vi "HyperTerm Data Decode.vi"(0 "Water Heater GEA2 Data in":T1 {"Hyperterminal Data"."CRC" format="%x"; "Hyperterminal Data"."Length" format="%x"; "Hyperterminal Data"."Command" format="%x"; "Hyperterminal Data"."Destination" format="%x"; "Hyperterminal Data"."Source" format="%x"}, 1 "Hex Array Out":string[](array[string]), 5 "Error In":errorcluster) -> (14 "Water Heater GEA2 Data out":T1 {"Hyperterminal Data"."CRC" format="%x"; "Hyperterminal Data"."Length" format="%x"; "Hyperterminal Data"."Command" format="%x"; "Hyperterminal Data"."Destination" format="%x"; "Hyperterminal Data"."Source" format="%x"}, 19 "Error Out":errorcluster)   [LabVIEW 2018]
uses:
  Type Definitions/GEA2 Commands WaterHeater GEA2 Data.ctl
  Type Definitions/GEA2 Commands Button Status.ctl
  Type Definitions/GEA2 Commands Status Query.ctl
  Type Definitions/GEA2 Commands Service Error Codes.ctl
panel:
  out "String":string
  out "T5(Ambient)":dbl
  out "T4(CompressorDischarge)":dbl
  out "T3B (EvapOut)":dbl
  out "T3A (EvapIN)":dbl
  out "T2 Tank Sensor":dbl
  out "Reason for Data Word 4":string
  out "Reason for Data Word 3":string
  out "Reason for Data Word 2":string
  out "Reason for Data Word 1":string
  out "Reason for last heating cycle termination":u16
  out "EEV Position (0-480)":u16
  out "Voltage (Volts)":u16
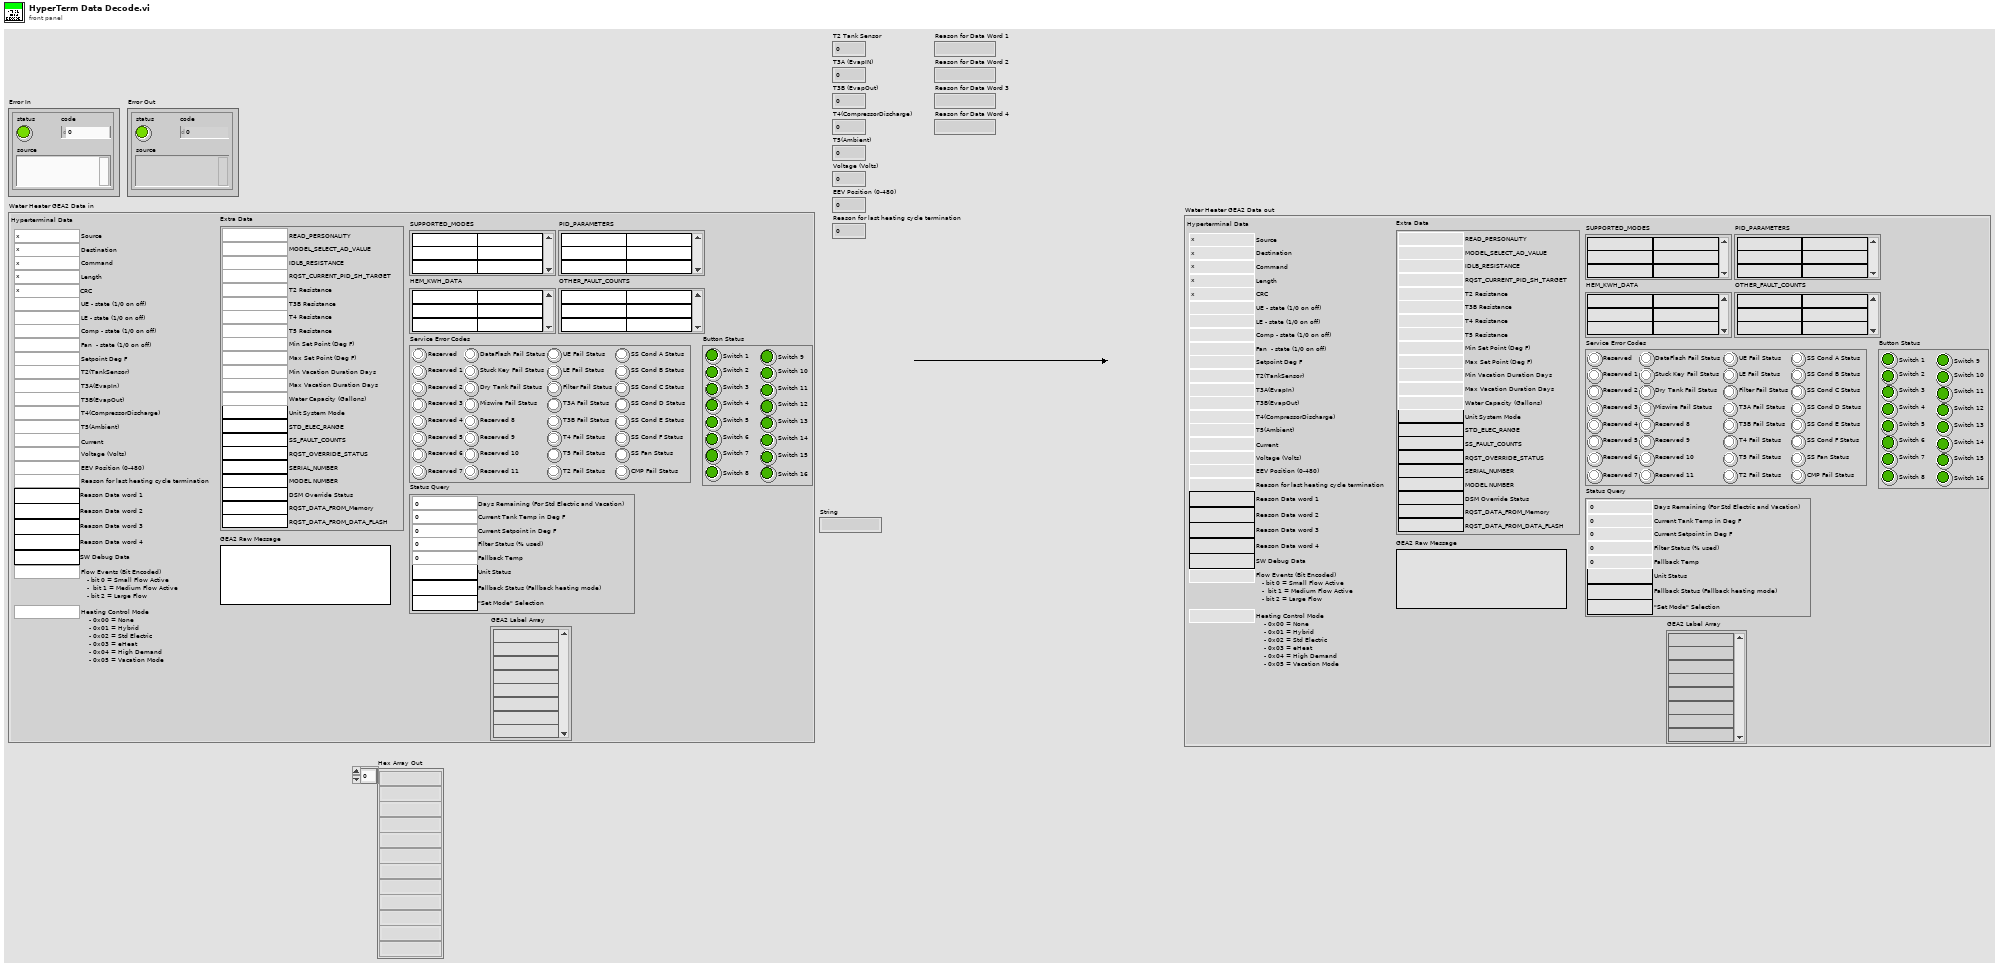
[diagram p1: front panel]
types:
  T1 = typedef "GEA2 Commands WaterHeater GEA2 Data.ctl" = cluster{"GEA2 Label Array":string[], "PID_PARAMETERS":string[][], "SUPPORTED_MODES":string[][], "Button Status":T2, "Status Query":T3, "Service Error Codes":T4, "HEM_KWH_DATA":string[][], "OTHER_FAULT_COUNTS":string[][], "GEA2 Raw Message":string, "Hyperterminal Data":cluster{"Source":u8, "Destination":u8, "Command":u8, "Length":u8, "CRC":u16, "UE - state (1/0 on off)":u8, "LE - state (1/0 on off)":u8, "Comp - state (1/0 on off)":u8, "Fan  - state (1/0 on off)":u8, "Setpoint Deg F":i32, "T2(TankSensor)":dbl, "T3A(EvapIn)":dbl, "T3B(EvapOut)":dbl, "T4(CompressorDischarge)":dbl, "T5(Ambient)":dbl, "Current":dbl, "Voltage (Volts)":u16, "EEV Position (0-480)":u16, "Reason for last heating cycle termination":u16, "Reason Data word 1":string, "Reason Data word 2":string, "Reason Data word 3":string, "Reason Data word 4":string, "SW Debug Data":string, "Flow Events (Bit Encoded)":u16, "Heating Control Mode":u16}, "Extra Data":cluster{"Water Capacity (Gallons)":u32, "Max Vacation Duration Days":u32, "Min Vacation Duration Days":u32, "Max Set Point (Deg F)":u32, "Min Set Point (Deg F)":u32, "T5 Resistance":u32, "T4 Resistance":u32, "T3B Resistance":u32, "T2 Resistance":u32, "STD_ELEC_RANGE":string, "SS_FAULT_COUNTS":string, "SERIAL_NUMBER":string, "READ_PERSONALITY":u8, "RQST_OVERRIDE_STATUS":string, "MODEL_SELECT_AD_VALUE":u32, "MODEL NUMBER":string, "IDLB_RESISTANCE":u32, "DSM Override Status":string, "RQST_DATA_FROM_Memory":string, "RQST_DATA_FROM_DATA_FLASH":string, "RQST_CURRENT_PID_SH_TARGET":u16, "Unit System Mode":string}}
  T2 = typedef "GEA2 Commands Button Status.ctl" = cluster{"Switch 1":bool, "Switch 2":bool, "Switch 3":bool, "Switch 4":bool, "Switch 5":bool, "Switch 6":bool, "Switch 7":bool, "Switch 8":bool, "Switch 9":bool, "Switch 10":bool, "Switch 11":bool, "Switch 12":bool, "Switch 13":bool, "Switch 14":bool, "Switch 15":bool, "Switch 16":bool}
  T3 = typedef "GEA2 Commands Status Query.ctl" = cluster{"Days Remaining (For Std Electric and Vacation)":u8, "Unit Status":string, "Current Tank Temp in Deg F":u8, "Current Setpoint in Deg F":u8, "Filter Status (% used)":u8, "Fallback Status (Fallback heating mode)":string, "Fallback Temp":u8, "\"Set Mode\" Selection":string}
  T4 = typedef "GEA2 Commands Service Error Codes.ctl" = cluster{"Reserved":bool, "Reserved 1":bool, "Reserved 2":bool, "Reserved 3":bool, "Reserved 4":bool, "Reserved 5":bool, "Reserved 6":bool, "Reserved 7":bool, "DataFlash Fail Status":bool, "Stuck Key Fail Status":bool, "Dry Tank Fail Status":bool, "Miswire Fail Status":bool, "Reserved 8":bool, "Reserved 9":bool, "Reserved 10":bool, "Reserved 11":bool, "UE Fail Status":bool, "LE Fail Status":bool, "Filter Fail Status":bool, "T3A Fail Status":bool, "T3B Fail Status":bool, "T4 Fail Status":bool, "T5 Fail Status":bool, "T2 Fail Status":bool, "SS Cond A Status":bool, "SS Cond B Status":bool, "SS Cond C Status":bool, "SS Cond D Status":bool, "SS Cond E Status":bool, "SS Cond F Status":bool, "SS Fan Status":bool, "CMP Fail Status":bool}
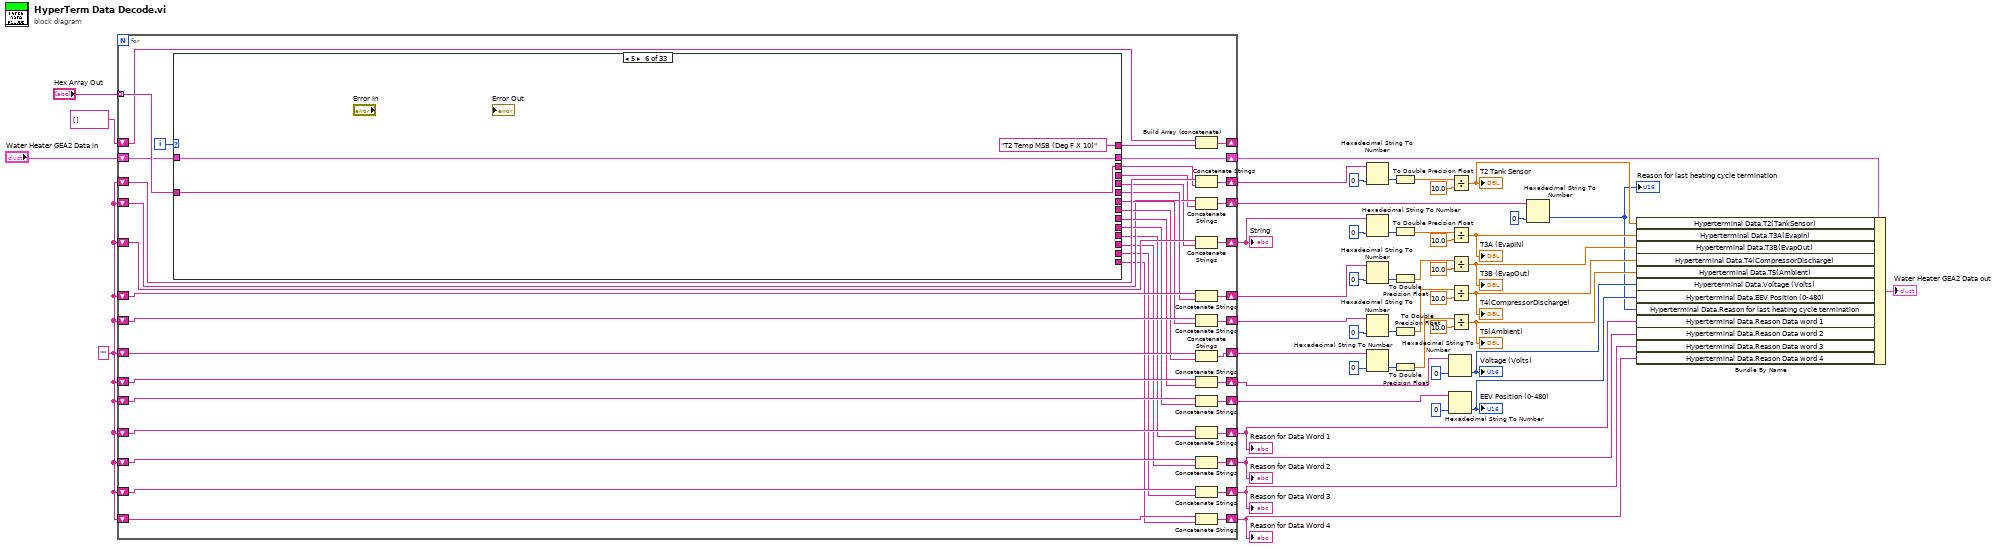
[diagram p0: block diagram]
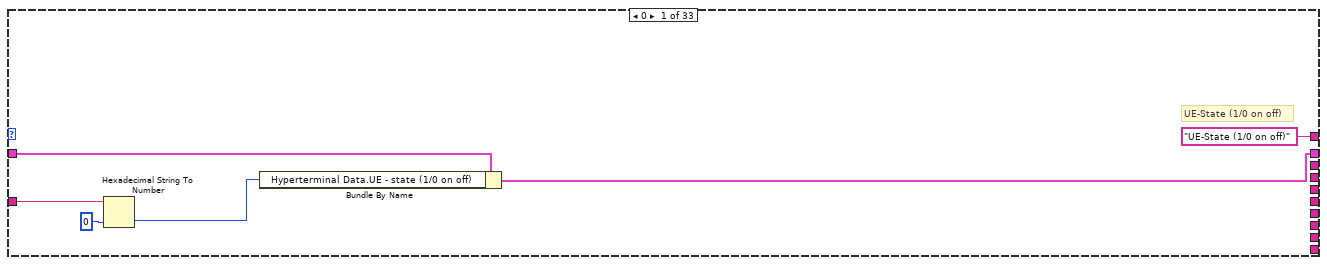
[diagram p2: hidden frame]
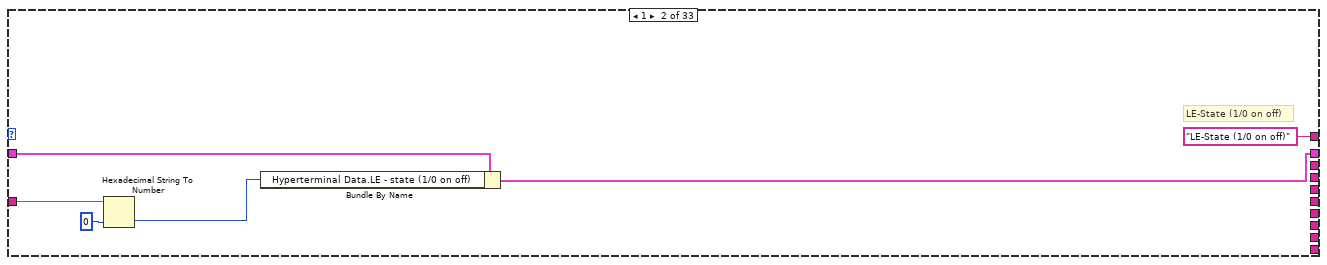
[diagram p3: hidden frame]
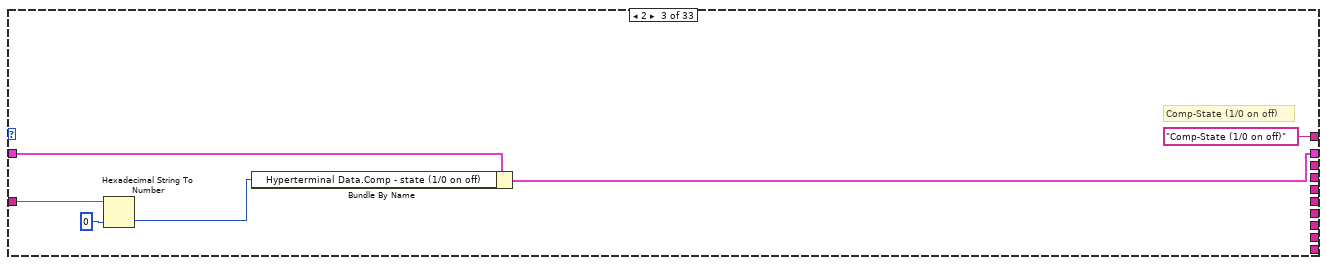
[diagram p4: hidden frame]
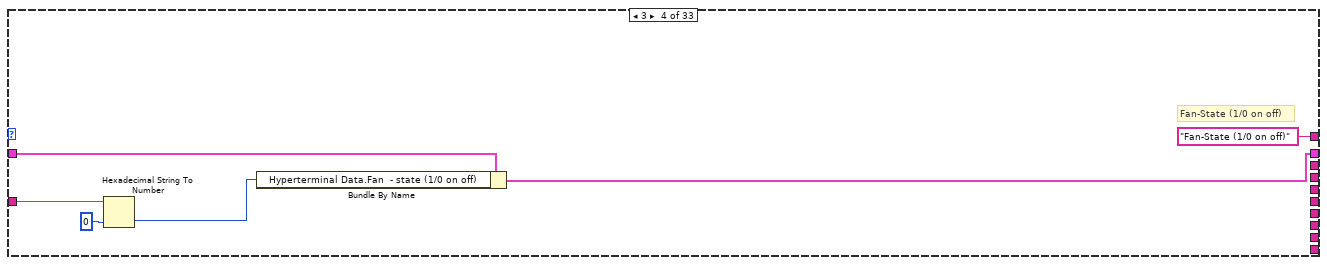
[diagram p5: hidden frame]
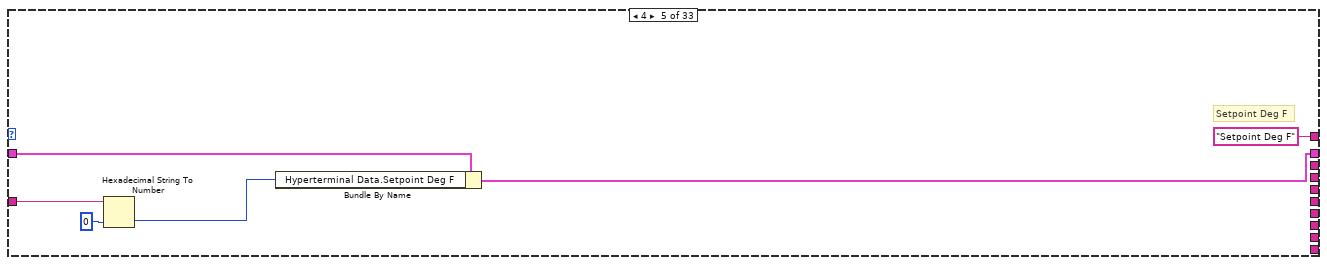
[diagram p6: hidden frame]
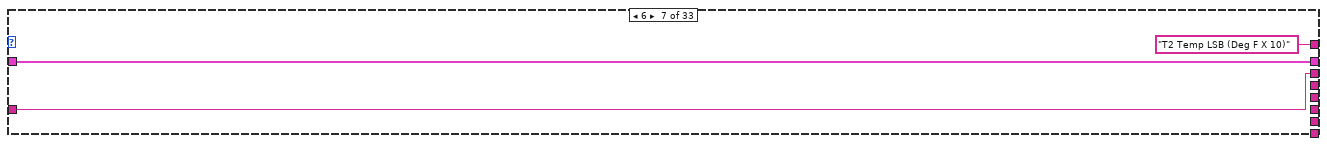
[diagram p7: hidden frame]
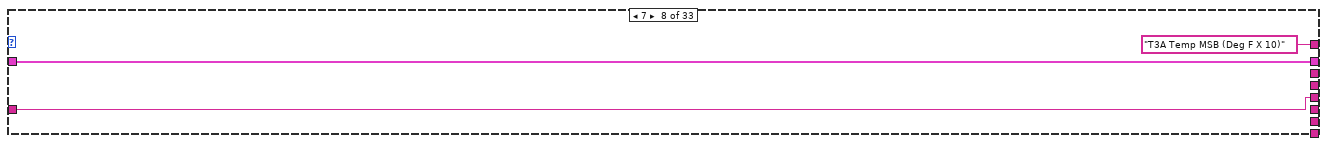
[diagram p8: hidden frame]
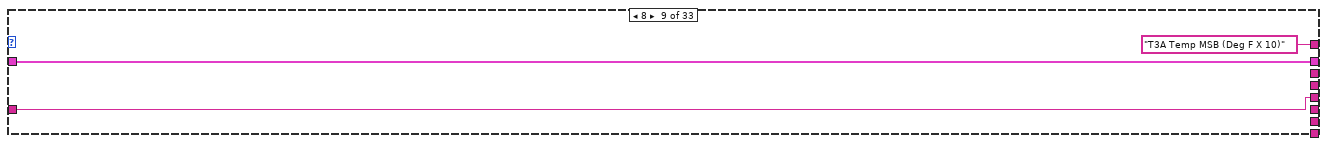
[diagram p9: hidden frame]
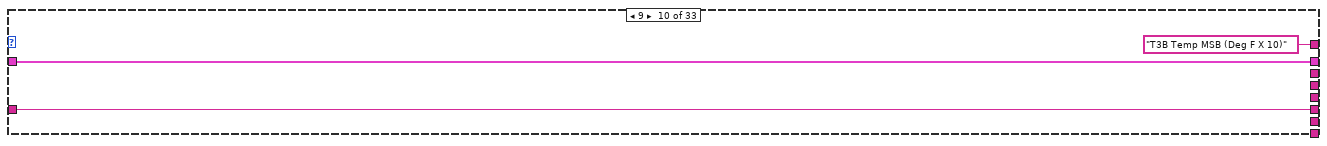
[diagram p10: hidden frame]
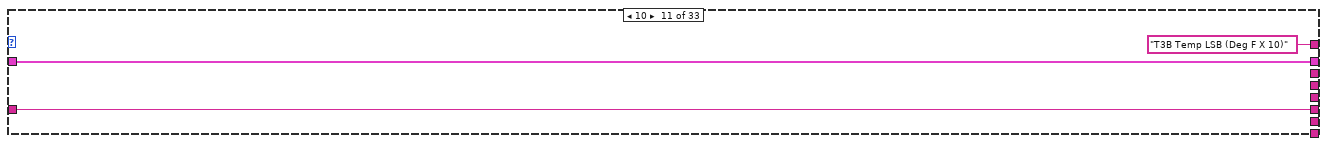
[diagram p11: hidden frame]
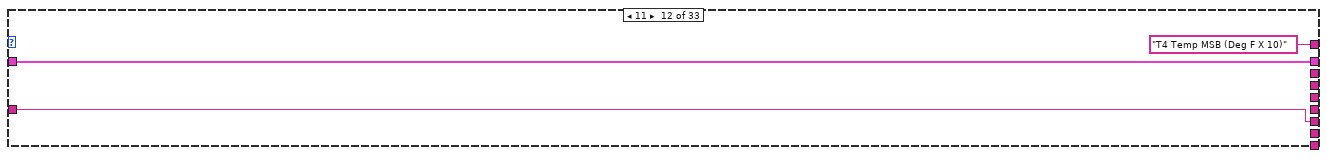
[diagram p12: hidden frame]
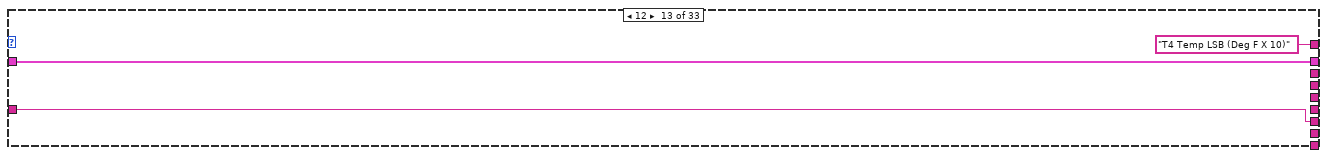
[diagram p13: hidden frame]
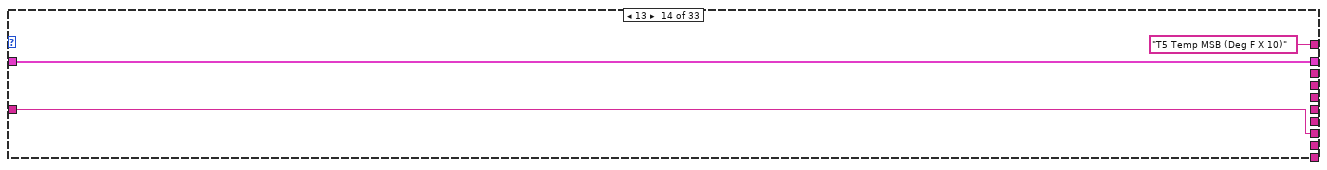
[diagram p14: hidden frame]
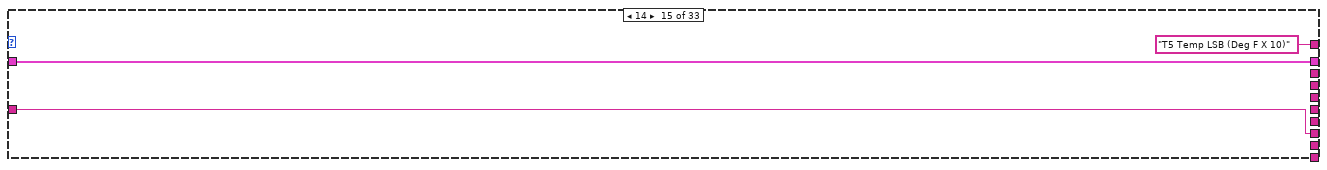
[diagram p15: hidden frame]
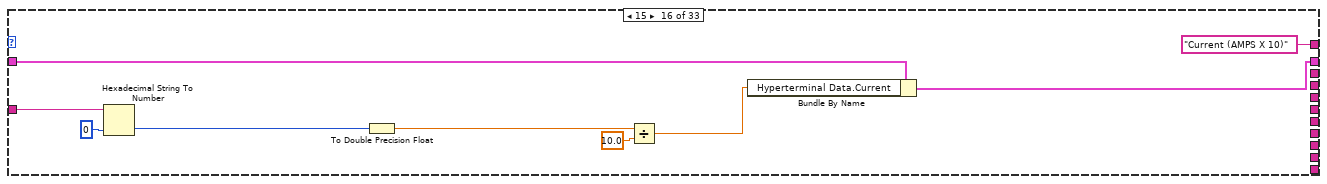
[diagram p16: hidden frame]
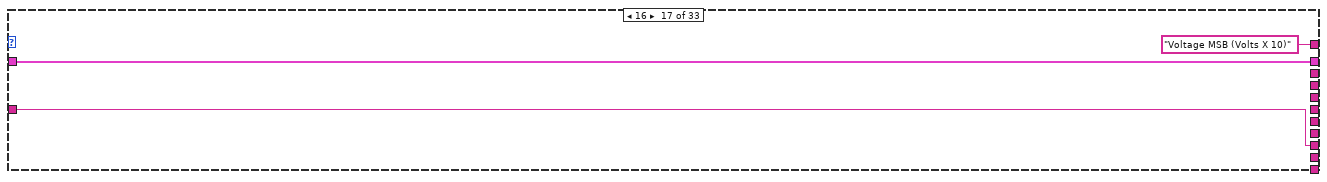
[diagram p17: hidden frame]
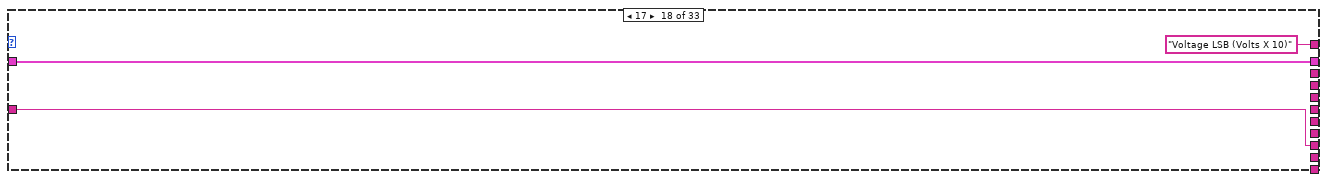
[diagram p18: hidden frame]
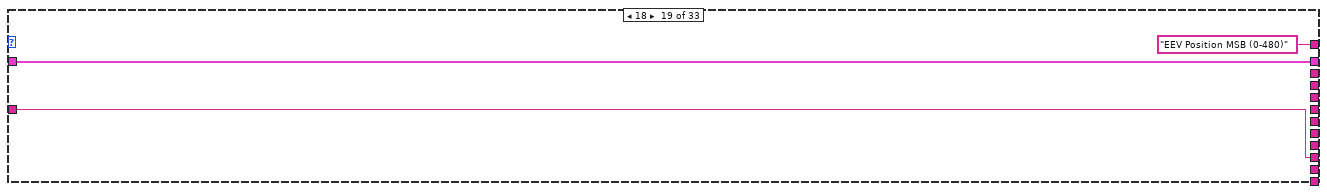
[diagram p19: hidden frame]
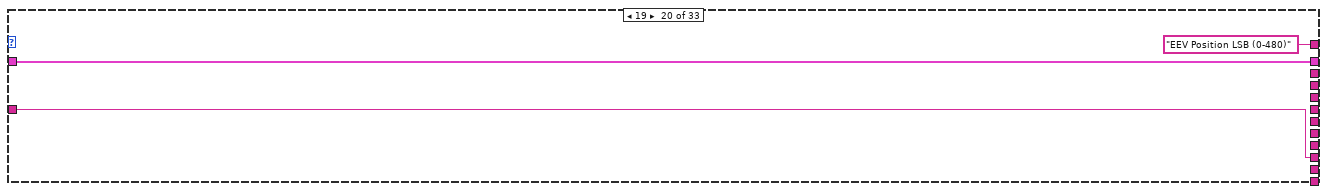
[diagram p20: hidden frame]
diagram:
  w47 = ""
  n1 = for {
    tunnel: "Hex Array Out" -> [w91] mode=indexing
    shift-right: [w88] -> _
    shift-left: string[] [] -> [w90]
    shift-right: [w84] -> w14
    shift-left: "Water Heater GEA2 Data in" -> [w85]
    shift-right: [w51] -> w45
    shift-left: w47 -> [w87]
    shift-right: [w82] -> w44
    shift-left: w47 -> [w83]
    shift-right: [w79] -> w43
    shift-left: w47 -> [w81]
    shift-right: [w76] -> w42
    shift-left: w47 -> [w78]
    shift-right: [w73] -> w41
    shift-left: w47 -> [w75]
    shift-right: [w70] -> w40
    shift-left: w47 -> [w72]
    shift-right: [w67] -> w39
    shift-left: w47 -> [w69]
    shift-right: [w64] -> w38
    shift-left: w47 -> [w66]
    shift-right: [w61] -> w4
    shift-left: w47 -> [w63]
    shift-right: [w58] -> w3
    shift-left: w47 -> [w60]
    shift-right: [w55] -> w2
    shift-left: w47 -> [w57]
    shift-right: [w52] -> w1
    shift-left: w47 -> [w54]
    i -> [w92]
    n2 = case shown="5" w92 {
      tunnel: w91 -> [w95 w99 w105 w111 w117 w123 w126 w130 w133 w136 w139 w142 w145 w148 w151 w157 w163 w166 w169 w172 w177 w183 w187 w190 w193 w196 w199 w202 w205 w208 w211 w214 w217]
      tunnel: ["UE-State (1/0 on off)" "LE-State (1/0 on off)" "Comp-State (1/0 on off)" "Fan-State (1/0 on off)" "Setpoint Deg F" "T2 Temp MSB (Deg F X 10)" "T2 Temp LSB (Deg F X 10)" "T3A Temp MSB (Deg F X 10)" "T3A Temp MSB (Deg F X 10)" "T3B Temp MSB (Deg F X 10)" "T3B Temp LSB (Deg F X 10)" "T4 Temp MSB (Deg F X 10)" "T4 Temp LSB (Deg F X 10)" "T5 Temp MSB (Deg F X 10)" "T5 Temp LSB (Deg F X 10)" "Current (AMPS X 10)" "Voltage MSB (Volts X 10)" "Voltage LSB (Volts X 10)" "EEV Position MSB (0-480)" "EEV Position LSB (0-480)" "\"Flow Events (Bit Encoded)\n   - bit 0 = Small Flow Active\n   -  bit 1 = Medium Flow Active\n   - bit 2 = Large Flow\"\n" "Heating Control Mode\n    - 0x00 = None\n    - 0x01 = Hybrid\n    - 0x02 = Std Electric\n    - 0x03 = eHeat\n    - 0x04 = High Demand\n    - 0x05 = Vacation Mode" "Reason for last heating cycle termination, MSB\n" "Reason for last heating cycle termination, LSB" "Reason Data word 1, MSB" "Reason Data word 1, LSB" "Reason Data word 2, MSB" "Reason Data word 2, LSB" "Reason Data word 3, MSB" "Reason Data word 3, LSB" "Reason Data word 4, MSB" "Reason Data word 4, LSB" "SW Debug Data"] -> w89
      tunnel: [_ _ _ _ _ w123 w126 _ _ _ _ _ _ _ _ _ _ _ _ _ _ _ _ _ _ _ _ _ _ _ _ _ _] -> w86
      tunnel: w85 -> [w97 w102 w108 w114 w118 w124 w127 w129 w132 w135 w138 w141 w144 w147 w150 w160 w162 w165 w168 w171 w176 w182 w186 w189 w192 w195 w198 w201 w204 w207 w210 w213 w219]
      tunnel: [w96 w101 w107 w113 w119 w124 w127 w129 w132 w135 w138 w141 w144 w147 w150 w159 w162 w165 w168 w171 w175 w181 w186 w189 w192 w195 w198 w201 w204 w207 w210 w213 w220] -> w84
      tunnel: [_ _ _ _ _ _ _ w130 w133 _ _ _ _ _ _ _ _ _ _ _ _ _ _ _ _ _ _ _ _ _ _ _ _] -> w50
      tunnel: [_ _ _ _ _ _ _ _ _ w136 w139 _ _ _ _ _ _ _ _ _ _ _ _ _ _ _ _ _ _ _ _ _ _] -> w80
      tunnel: [_ _ _ _ _ _ _ _ _ _ _ w142 w145 _ _ _ _ _ _ _ _ _ _ _ _ _ _ _ _ _ _ _ _] -> w77
      tunnel: [_ _ _ _ _ _ _ _ _ _ _ _ _ w148 w151 _ _ _ _ _ _ _ _ _ _ _ _ _ _ _ _ _ _] -> w74
      tunnel: [_ _ _ _ _ _ _ _ _ _ _ _ _ _ _ _ w163 w166 _ _ _ _ _ _ _ _ _ _ _ _ _ _ _] -> w71
      tunnel: [_ _ _ _ _ _ _ _ _ _ _ _ _ _ _ _ _ _ w169 w172 _ _ _ _ _ _ _ _ _ _ _ _ _] -> w68
      tunnel: [_ _ _ _ _ _ _ _ _ _ _ _ _ _ _ _ _ _ _ _ _ _ w187 w190 _ _ _ _ _ _ _ _ _] -> w65
      tunnel: [_ _ _ _ _ _ _ _ _ _ _ _ _ _ _ _ _ _ _ _ _ _ _ _ w193 w196 _ _ _ _ _ _ _] -> w62
      tunnel: [_ _ _ _ _ _ _ _ _ _ _ _ _ _ _ _ _ _ _ _ _ _ _ _ _ _ w199 w202 _ _ _ _ _] -> w59
      tunnel: [_ _ _ _ _ _ _ _ _ _ _ _ _ _ _ _ _ _ _ _ _ _ _ _ _ _ _ _ w205 w208 _ _ _] -> w56
      tunnel: [_ _ _ _ _ _ _ _ _ _ _ _ _ _ _ _ _ _ _ _ _ _ _ _ _ _ _ _ _ _ w211 w214 _] -> w53
      frame 0 {
        # "UE-State (1/0 on off)"
        n3 = Hexadecimal String To Number(string=w95, default (0uL)=u8 0 ("default (0 U32)")) -> (number=w93:u8)  [unwired: 1 in, 1 out]
        n4 = Bundle By Name(cluster=w97, "Hyperterminal Data.UE - state (1/0 on off)"=w93) -> (w96:T1)
      }
      frame 1 {
        # "LE-State (1/0 on off)"
        n5 = Hexadecimal String To Number(string=w99, default (0uL)=u8 0 ("default (0 U32)")) -> (number=w100:u8)  [unwired: 1 in, 1 out]
        n6 = Bundle By Name(cluster=w102, "Hyperterminal Data.LE - state (1/0 on off)"=w100) -> (w101:T1)
      }
      frame 2 {
        # "Comp-State (1/0 on off)"
        n7 = Hexadecimal String To Number(string=w105, default (0uL)=u8 0 ("default (0 U32)")) -> (number=w106:u8)  [unwired: 1 in, 1 out]
        n8 = Bundle By Name(cluster=w108, "Hyperterminal Data.Comp - state (1/0 on off)"=w106) -> (w107:T1)
      }
      frame 3 {
        # "Fan-State (1/0 on off)"
        n9 = Hexadecimal String To Number(string=w111, default (0uL)=u8 0 ("default (0 U32)")) -> (number=w112:u8)  [unwired: 1 in, 1 out]
        n10 = Bundle By Name(cluster=w114, "Hyperterminal Data.Fan  - state (1/0 on off)"=w112) -> (w113:T1)
      }
      frame 4 {
        # "Setpoint Deg F"
        n11 = Hexadecimal String To Number(string=w117, default (0uL)=0 ("default (0 U32)")) -> (number=w120:i32)  [unwired: 1 in, 1 out]
        n12 = Bundle By Name(cluster=w118, "Hyperterminal Data.Setpoint Deg F"=w120) -> (w119:T1)
      }
      frame 5 {
      }
      frame 6 {
      }
      frame 7 {
      }
      frame 8 {
      }
      frame 9 {
      }
      frame 10 {
      }
      frame 11 {
      }
      frame 12 {
      }
      frame 13 {
      }
      frame 14 {
      }
      frame 15 {
        n13 = Hexadecimal String To Number(string=w157, default (0uL)=u16 0 ("default (0 U32)")) -> (number=w154:u16)  [unwired: 1 in, 1 out]
        n14 = To Double Precision Float(number=w154) -> (double precision float=w155:dbl)
        n15 = Divide(x=w155, y=10.0) -> (x/y=w153:dbl)
        n16 = Bundle By Name(cluster=w160, "Hyperterminal Data.Current"=w153) -> (w159:T1)
      }
      frame 16 {
      }
      frame 17 {
      }
      frame 18 {
      }
      frame 19 {
      }
      frame 20 {
        n17 = Hexadecimal String To Number(string=w177, default (0uL)=u16 0 ("default (0 U32)")) -> (number=w174:u16)  [unwired: 1 in, 1 out]
        n18 = Bundle By Name(cluster=w176, "Hyperterminal Data.Flow Events (Bit Encoded)"=w174) -> (w175:T1)
      }
      frame 21 {
        n19 = Hexadecimal String To Number(string=w183, default (0uL)=u16 0 ("default (0 U32)")) -> (number=w180:u16)  [unwired: 1 in, 1 out]
        n20 = Bundle By Name(cluster=w182, "Hyperterminal Data.Heating Control Mode"=w180) -> (w181:T1)
      }
      frame 22 {
      }
      frame 23 {
      }
      frame 24 {
      }
      frame 25 {
      }
      frame 26 {
      }
      frame 27 {
      }
      frame 28 {
      }
      frame 29 {
      }
      frame 30 {
      }
      frame 31 {
      }
      frame 32, Default {
        n21 = Unbundle By Name(w219) -> ("Hyperterminal Data.SW Debug Data"=w218:string)
        n22 = Concatenate Strings(w218, w217) -> (w216:string)
        n23 = Bundle By Name(cluster=w219, "Hyperterminal Data.SW Debug Data"=w216) -> (w220:T1)
      }
    }
    n24 = Build Array (concatenate)(w90, w89) -> (w88:string[])
    n25 = Concatenate Strings(w87, w86) -> (w51:string)
    n26 = Concatenate Strings(w66, w65) -> (w64:string)
    n27 = Concatenate Strings(w83, w50) -> (w82:string)
    n28 = Concatenate Strings(w81, w80) -> (w79:string)
    n29 = Concatenate Strings(w78, w77) -> (w76:string)
    n30 = Concatenate Strings(w75, w74) -> (w73:string)
    n31 = Concatenate Strings(w72, w71) -> (w70:string)
    n32 = Concatenate Strings(w69, w68) -> (w67:string)
    n33 = Concatenate Strings(w63, w62) -> (w61:string)
    n34 = Concatenate Strings(w60, w59) -> (w58:string)
    n35 = Concatenate Strings(w57, w56) -> (w55:string)
    n36 = Concatenate Strings(w54, w53) -> (w52:string)
  }
  "Reason for Data Word 1" <- w4
  "Reason for Data Word 2" <- w3
  "Reason for Data Word 3" <- w2
  "Reason for Data Word 4" <- w1
  "String" <- w44
  n37 = Hexadecimal String To Number(string=w45, default (0uL)=u16 0) -> (number=w28:u16)  [unwired: 1 in, 1 out]
  n38 = Hexadecimal String To Number(string=w44, default (0uL)=u16 0) -> (number=w24:u16)  [unwired: 1 in, 1 out]
  n39 = Hexadecimal String To Number(string=w43, default (0uL)=u16 0) -> (number=w21:u16)  [unwired: 1 in, 1 out]
  n40 = Hexadecimal String To Number(string=w42, default (0uL)=u16 0) -> (number=w18:u16)  [unwired: 1 in, 1 out]
  n41 = Hexadecimal String To Number(string=w41, default (0uL)=u16 0) -> (number=w15:u16)  [unwired: 1 in, 1 out]
  n42 = To Double Precision Float(number=w28) -> (double precision float=w27:dbl)
  n43 = To Double Precision Float(number=w24) -> (double precision float=w26:dbl)
  n44 = To Double Precision Float(number=w21) -> (double precision float=w22:dbl)
  n45 = To Double Precision Float(number=w18) -> (double precision float=w20:dbl)
  n46 = To Double Precision Float(number=w15) -> (double precision float=w16:dbl)
  n47 = Hexadecimal String To Number(string=w40, default (0uL)=u16 0) -> (number=w7:u16)  [unwired: 1 in, 1 out]
  "Voltage (Volts)" <- w7
  n48 = Hexadecimal String To Number(string=w39, default (0uL)=u16 0) -> (number=w6:u16)  [unwired: 1 in, 1 out]
  "EEV Position (0-480)" <- w6
  n49 = Divide(x=w27, y=10.0) -> (x/y=w13:dbl)
  "T2 Tank Sensor" <- w13
  n50 = Divide(x=w26, y=10.0) -> (x/y=w11:dbl)
  "T3A (EvapIN)" <- w11
  n51 = Divide(x=w22, y=10.0) -> (x/y=w10:dbl)
  "T3B (EvapOut)" <- w10
  n52 = Divide(x=w20, y=10.0) -> (x/y=w9:dbl)
  "T4(CompressorDischarge)" <- w9
  n53 = Divide(x=w16, y=10.0) -> (x/y=w8:dbl)
  "T5(Ambient)" <- w8
  n54 = Hexadecimal String To Number(string=w38, default (0uL)=u16 0) -> (number=w5:u16)  [unwired: 1 in, 1 out]
  "Reason for last heating cycle termination" <- w5
  n55 = Bundle By Name(cluster=w14, "Hyperterminal Data.T2(TankSensor)"=w13, "Hyperterminal Data.T3A(EvapIn)"=w11, "Hyperterminal Data.T3B(EvapOut)"=w10, "Hyperterminal Data.T4(CompressorDischarge)"=w9, "Hyperterminal Data.T5(Ambient)"=w8, "Hyperterminal Data.Voltage (Volts)"=w7, "Hyperterminal Data.EEV Position (0-480)"=w6, "Hyperterminal Data.Reason for last heating cycle termination"=w5, "Hyperterminal Data.Reason Data word 1"=w4, "Hyperterminal Data.Reason Data word 2"=w3, "Hyperterminal Data.Reason Data word 3"=w2, "Hyperterminal Data.Reason Data word 4"=w1) -> (→"Water Heater GEA2 Data out":T1)
